vi "SECoP_dataCompare.vi"(8 "error in (no error)":errorcluster, 9 "SECoP_dataPtr (2)":T2 {"ptr64" format="%.0x"; "ptr32" format="%.0x"}, 10 "SECoP_dataPtr (1)":T2 {"ptr64" format="%.0x"; "ptr32" format="%.0x"}, 11 "DLL path (in)":T3) -> (0 "error out":errorcluster, 2 "compare result":T1, 3 "DLL path (out)":T3)   [LabVIEW 2023, in "SECoP.lvlib"]
doc: "Call <b>\"SECoP_dataCompare.vi\"</b> to compare two \"SECoP-data.ctl\" values (SECoP_dataPtr).\n\n<b>DLL path</b> input and output of cluster from \"SECoP-Initialize.vi\"\n<b>SECoP_dataPtr (1)</b> first value to compare\n<b>SECoP_dataPtr (2)</b> second value to compare\n<b>compare result</b> result could be equal, similar or different in value or type (see \"SECoP-data.ctl\")"
uses:
  SECoP.lvlib
  SECoP-libraries.ctl
  SECoP-data.ctl
  SECoP-dataCompareResult.ctl
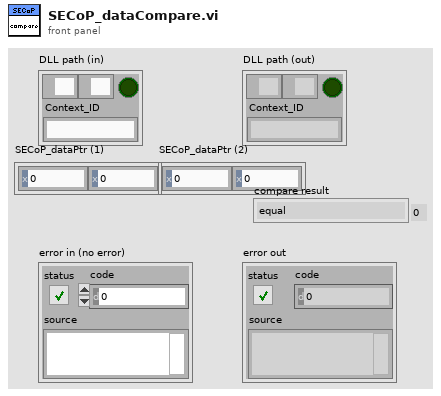
[diagram p1: front panel]
types:
  T1 = typedef "SECoP.lvlib/SECoP-dataCompareResult.ctl" = enum32{"equal", "similar value", "different value", "different type"}
  T2 = typedef "SECoP.lvlib/SECoP-data.ctl" = cluster{"ptr32":u32, "ptr64":u64}
  T3 = typedef "SECoP.lvlib/SECoP-libraries.ctl" = cluster{"serverDLL":path, "variantDLL":path, "cleanup_mode":bool, "Context_ID":string}
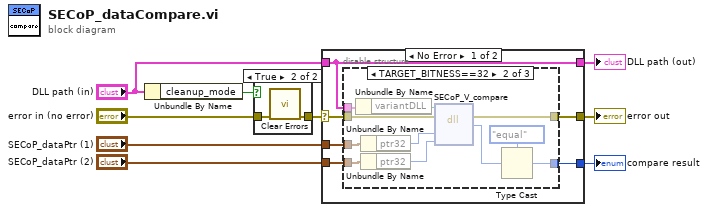
[diagram p0: block diagram]
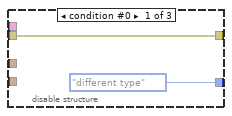
[diagram p3: hidden frame]
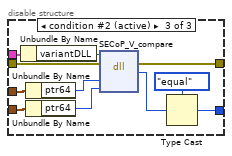
[diagram p4: hidden frame]
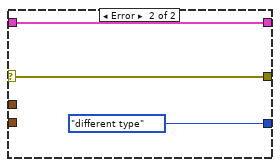
[diagram p5: hidden frame]
diagram:
  n1 = Unbundle By Name("DLL path (in)") -> ("cleanup_mode"=w7:bool)
  n2 = case shown="True" w7 {
    tunnel: "error in (no error)" -> [w10 w12]
    tunnel: [w10 w11] -> w5
    frame False {
    }
    frame True {
      n3 = call <vilib>:"Clear Errors.vi"("error in (no error)"=w12) -> ("error out"=w11:errorcluster)  [unwired: 5 in, 1 out]
    }
  }
  n4 = case shown="No Error" w5 {
    selector: w5 -> [w17 w44]
    tunnel: "DLL path (in)" -> [w13 w45]
    tunnel: [w13 w45] -> w9
    tunnel: [w15 w44] -> w8
    tunnel: "SECoP_dataPtr (1)" -> [w18 _]
    tunnel: "SECoP_dataPtr (2)" -> [w16 _]
    tunnel: [w14 SECoP-dataCompareResult."different type" ("compare result")] -> w1
    frame No Error {
      n5 = disable-structure shown="TARGET_BITNESS==32" {
        disable-tunnel: w18 -> [_ w28 w39]
        disable-tunnel: w17 -> [w20 w31 w42]
        disable-tunnel: w13 -> [_ w30 w41]
        disable-tunnel: [w20 w29 w40] -> w15
        disable-tunnel: w16 -> [_ w27 w38]
        disable-tunnel: [SECoP-dataCompareResult."different type" ("compare result") w22 w33] -> w14
        frame condition #0 {
        }
        frame condition #1 {
          n6 = Unbundle By Name(w30) -> ("variantDLL"=w21:path)
          n7 = Unbundle By Name(w28) -> ("ptr32"=w26:u32)
          n8 = Unbundle By Name(w27) -> ("ptr32"=w25:u32)
          n9 = dll-call lib="Z:/Praktische_Aufgaben/SECoP-LabVIEW2015/32bit/SECoP32.dll" fn="SECoP_V_compare"(path in=w21, error in=w31, "pData1"=w26, "pData2"=w25) -> (error out=w29:errorcluster, "return type"=w24:i32)  [unwired: 3 in, 1 out]
          n10 = Type Cast(type=SECoP-dataCompareResult."equal" ("compare result"), x=w24) -> (*(type *) &x=w22:T1)
        }
        frame condition #2 (active) {
          n11 = Unbundle By Name(w41) -> ("variantDLL"=w32:path)
          n12 = Unbundle By Name(w39) -> ("ptr64"=w37:u64)
          n13 = Unbundle By Name(w38) -> ("ptr64"=w36:u64)
          n14 = dll-call lib="Z:/Praktische_Aufgaben/SECoP-LabVIEW2015/32bit/SECoP32.dll" fn="SECoP_V_compare"(path in=w32, error in=w42, "pData1"=w37, "pData2"=w36) -> (error out=w40:errorcluster, "return type"=w35:i32)  [unwired: 3 in, 1 out]
          n15 = Type Cast(type=SECoP-dataCompareResult."equal" ("compare result"), x=w35) -> (*(type *) &x=w33:T1)
        }
      }
    }
    frame Error {
    }
  }
  "DLL path (out)" <- w9
  "error out" <- w8
  "compare result" <- w1
